vi "NewDeviceDetected.vi"(10 "Serial Number":string) -> (2 "Ignore?":bool, 3 "Selected Side":string(combo)="Right")   [LabVIEW 2013, in "main.lvlib"]
uses:
  main.lvlib
panel:
  in  "Ignore":bool
  in  "Save":bool
  in  "Side":string(combo)="Right"
  out "NewDeviceMsg":string
  # "Nyt Bluetooth apparat er blevet opdaget"
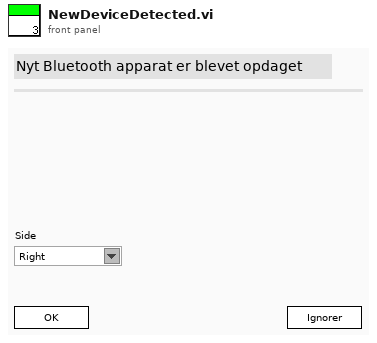
[diagram p1: front panel]
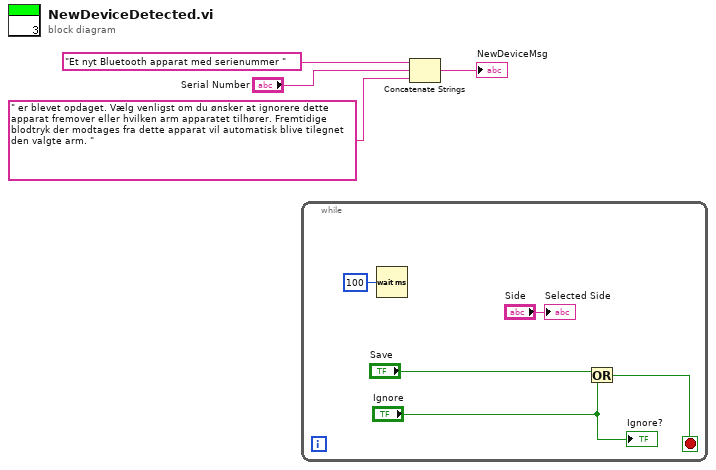
[diagram p0: block diagram]
diagram:
  n1 = while {
    stop <- w7 stop-if-true
    n2 = Wait (ms)(milliseconds to wait=u32 100) -> ()  [unwired: 1 out]
    n3 = Or(x="Save", y="Ignore") -> (x .or. y?=w7:bool)
    "Ignore?" <- "Ignore"
    "Selected Side" <- "Side"
  }
  n4 = Concatenate Strings("Et nyt Bluetooth apparat med serienummer ", "Serial Number", " er blevet opdaget. Vælg venligst om du ønsker at ignorere dette apparat fremover eller hvilken arm apparatet tilhører. Fremtidige blodtryk der modtages fra dette apparat vil automatisk blive tilegnet den valgte arm. ") -> (→"NewDeviceMsg":string)
